vi "Read Displays.vi"(9 "NumericWithScale in":refnum<class "NumericWithScale.lvclass">) -> (3 "NumericWithScale out":refnum<class "NumericWithScale.lvclass">, 4 "Displays":refnum<class "Digital.lvclass">[](array[class]))   [LabVIEW 2014, in "NumericWithScale.lvclass"]
uses:
  NumericWithScale.lvclass
  Digital/Digital.lvclass
  NumericWithScale.lvclass/NumericWithScale.ctl
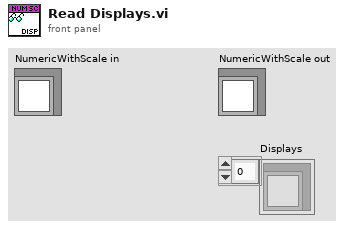
[diagram p1: front panel]
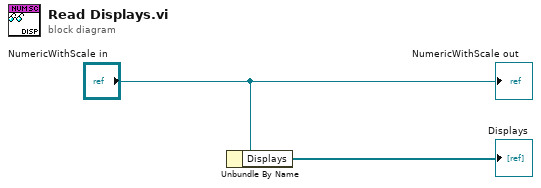
[diagram p0: block diagram]
diagram:
  n1 = Unbundle By Name("NumericWithScale in") -> ("Displays"=→"Displays":refnum<class "Digital.lvclass">[])
  "NumericWithScale out" <- "NumericWithScale in"
